vi "Data 2 Snapshot.vi"(9 "Snapshot Label":string, 11 "Data":dbl[](array[numeric])) -> (2 "Record":string)   [LabVIEW 2009]
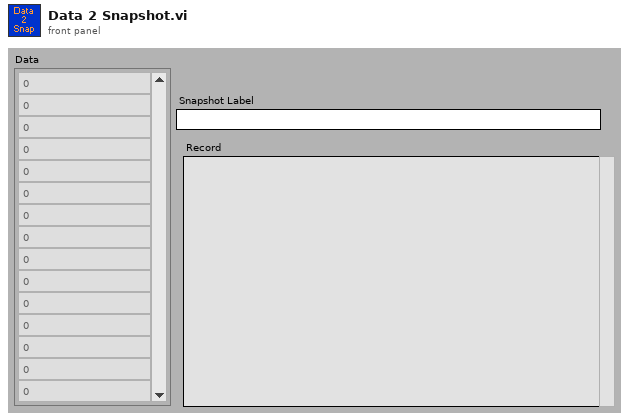
[diagram p1: front panel]
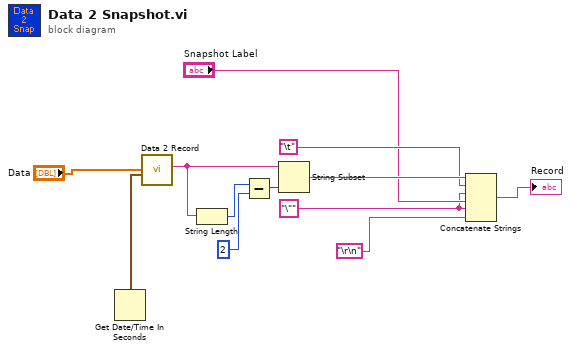
[diagram p0: block diagram]
diagram:
  w4 = "\""
  n1 = Get Date/Time In Seconds() -> (seconds since 1Jan1904=w12:timestamp)
  n2 = call "Data 2 Record.vi"("Time Stamp"=w12, "Data"="Data") -> ("Records"=w11:string)  [unwired: 1 in, 8 out]
  n3 = String Length(string=w11) -> (length=w3:i32)
  n4 = Subtract(x=w3, y=2) -> (x-y=w10:i32)
  n5 = String Subset(string=w11, length (rest)=w10) -> (substring=w9:string)  [unwired: 1 in]
  n6 = Concatenate Strings(w9, "\t", w4, "Snapshot Label", w4, "\r\n") -> (→"Record":string)
